vi "Set Osc Sample.vi"(8 "error in (no error)":errorcluster, 11 "sample":u32) -> (0 "error out":errorcluster, 3 "function return":u32)   [LabVIEW 2021, in "vmmsolib.lvlib"]
doc: "DLL_API unsigned int WINAPI SetOscSample(unsigned int sample);"
uses:
  vmmsolib.lvlib
  vmmso.dll
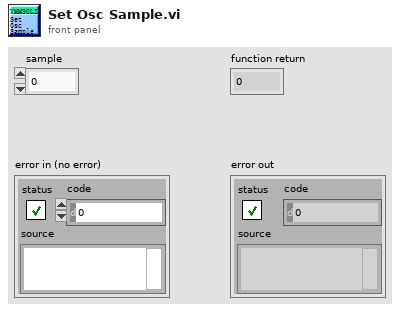
[diagram p1: front panel]
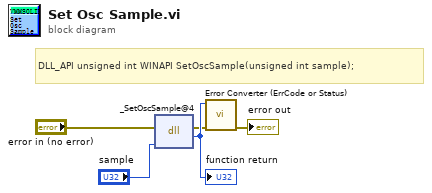
[diagram p0: block diagram]
diagram:
  # "DLL_API unsigned int WINAPI SetOscSample(unsigned int sample);"
  n1 = dll-call lib="D:/VmMsoSDK/demo-Labview/2021/vmmsolib/vmmso.*" fn="_SetOscSample@4"(error in="error in (no error)", "sample"="sample") -> (error out=w2:errorcluster, w5:u32)  [unwired: 3 in, 1 out]
  "function return" <- w5
  n2 = call "Error Converter (ErrCode or Status).vi"("error in (no error)"=w2, "error code"=w5) -> ("error out"=→"error out":errorcluster)  [unwired: 9 in]
